vi "Set Environment Variable.vi"(8 "Error In":errorcluster, 9 "Value":string, 10 "Name":string, 11 "Channel In":refnum<class "Channel.lvclass">) -> (0 "Error Out":errorcluster, 3 "Channel Out":refnum<class "Channel.lvclass">)   [LabVIEW 2018, in "Toolkit.lvlib" / "Channel.lvclass"]
uses:
  Channel.lvclass
  Channel.lvclass/Channel.ctl
  Session/Session.lvclass/Session.ctl
  SSH/SSH.lvclass/SSH.ctl
  Session/Session.lvclass
  Toolkit.lvlib
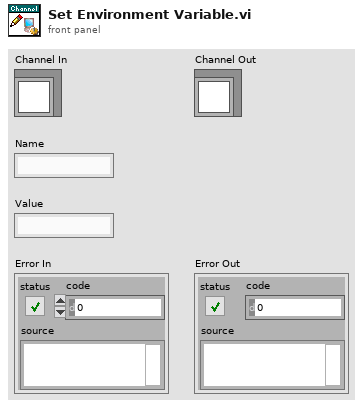
[diagram p1: front panel]
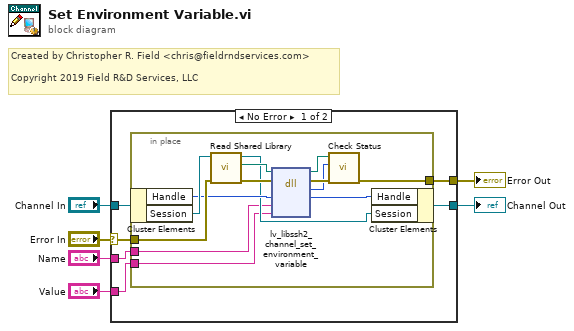
[diagram p0: block diagram]
diagram:
  # "Created by Christopher R. Field <chris@fieldrndservices.com>\n\nCopyright 2019 Field R&D Services, LLC"
  n1 = case shown="No Error" "Error In" {
    selector: "Error In" -> [w10 w27]
    tunnel: [w9 w27] -> w5
    tunnel: "Channel In" -> [w12 w26]
    tunnel: [w11 w26] -> w3
    tunnel: "Name" -> [w8 _]
    tunnel: "Value" -> [w7 _]
    frame No Error {
      n2 = in-place {
        in-place-border: w10 -> [w22]
        in-place-border: [w18] -> w9
        in-place-border: w8 -> [w14]
        in-place-border: w7 -> [w13]
        n3 = in-place-cluster #1(w12) -> ("Handle"=w17:u64, "Session"=w25:refnum<class "Session.lvclass">)
        n4 = call "Read Shared Library.vi"("Error In"=w22, "Session In"=w25) -> ("Erorr Out"=w23:errorcluster, "libssh2lv Shared Library"=w24:path, "Session Out"=w15:refnum<class "Session.lvclass">)  [unwired: 7 in]
        n5 = dll-call lib="libssh2lv.*" fn="lv_libssh2_channel_set_environment_variable"(path in=w24, error in=w23, "handle"=w17, "name"=w14, "value"=w13) -> (path out=w20:path, error out=w21:errorcluster, "status"=w19:i32, "handle"=w16:u64)  [unwired: 3 in]
        n6 = call "Check Status.vi"("Error In"=w21, "Status"=w19, "lv-libssh2 Shared Library In"=w20) -> ("Error Out"=w18:errorcluster)  [unwired: 7 in, 1 out]
        n7 = in-place-cluster #1("Handle"=w16, "Session"=w15) -> (w11:refnum<class "Channel.lvclass">)
      }
    }
    frame Error {
    }
  }
  "Error Out" <- w5
  "Channel Out" <- w3
